vi "FM_Rx_2012_.vi"() -> ()   [LabVIEW 2014]
uses:
  <instrlib>/niUSRP/niUSRP Fetch Rx Data (CDB WDT).vi
  <vilib>/Analysis/3filter.llb/FIR Filter (DBL).vi
  <vilib>/Analysis/3filter.llb/Butterworth Filter (DBL).vi
  <vilib>/Analysis/NI_AALPro.lvlib
  <vilib>/Analysis/NI_AALBase.lvlib
panel:
  out "Demodulated Output":waveform(dbl)(graph)
  in  "stop":bool
  out "error out":errorcluster
  in  "number of samples":i64=200000
  in  "active antenna":string="RX2"
  out "actual gain (dB)":dbl format="%#_6f"
  in  "gain (dB)":dbl format="%#_6f"
  out "actual carrier frequency":dbl=100000.0 format="%#_6p"
  in  "carrier frequency":dbl=915000000.0 format="%#_6p"
  out "actual IQ rate":dbl=100000.0 format="%#_6p"
  in  "IQ rate":dbl=1000000.0 format="%#_6p"
  in  "device names":refnum<k15>="192.168.10.2"
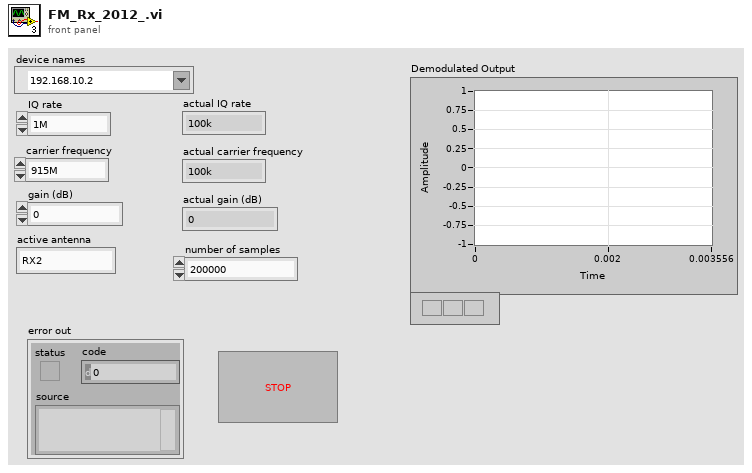
[diagram p1: front panel]
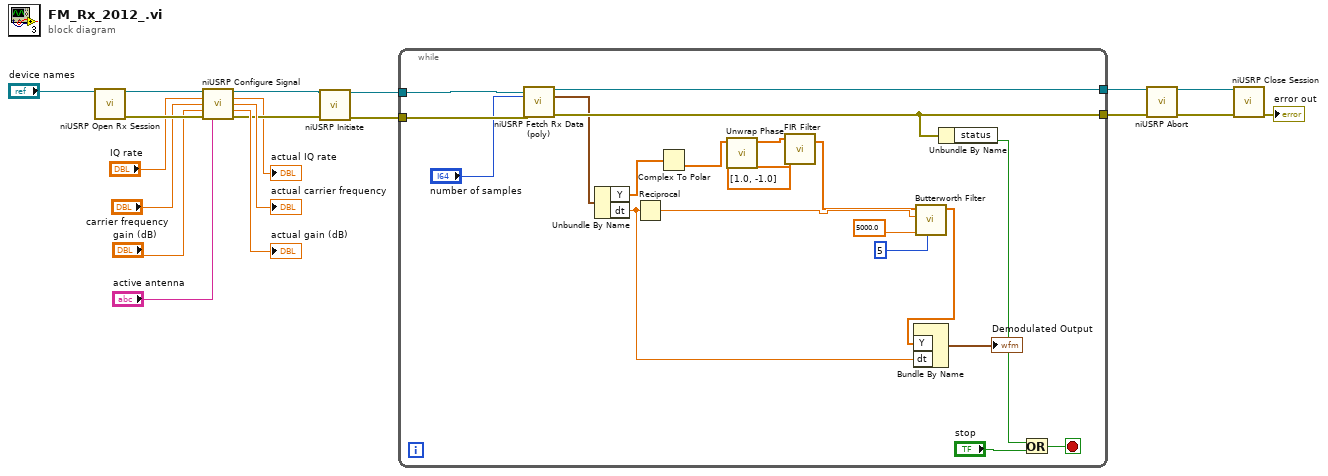
[diagram p0: block diagram]
diagram:
  n1 = call <instrlib>:"niUSRP Open Rx Session.vi"("device names"="device names") -> ("session handle out"=w18:refnum<k15>, "error out"=w17:errorcluster)  [unwired: 13 in]
  n2 = call <instrlib>:"niUSRP Configure Signal.vi"("session handle"=w18, "IQ rate"="IQ rate", "carrier frequency"="carrier frequency", "gain"="gain (dB)", "error in (no error)"=w17, "active antenna"="active antenna") -> ("session handle out"=w11:refnum<k15>, "coerced IQ rate"=→"actual IQ rate":dbl, "coerced carrier frequency"=→"actual carrier frequency":dbl, "coerced gain"=→"actual gain (dB)":dbl, "error out"=w10:errorcluster)  [unwired: 5 in]
  n3 = call <instrlib>:"niUSRP Initiate.vi"("session handle"=w11, "error in (no error)"=w10) -> ("session handle out"=w8:refnum<k15>, "error out"=w7:errorcluster)  [unwired: 12 in]
  n4 = while {
    tunnel: w8 -> [w39]
    tunnel: w7 -> [w38]
    tunnel: [w37] -> w6
    tunnel: [w33] -> w5
    stop <- w36 stop-if-true
    n5 = call-poly <instrlib>:"niUSRP Fetch Rx Data (poly).vi"("session handle"=w39, "number of samples"="number of samples", "error in (no error)"=w38) -> ("session handle out"=w37:refnum<k15>, "data"=w31:waveform(cdb), "error out"=w33:errorcluster)  [unwired: 9 in, 1 out]
    n6 = Unbundle By Name(w31) -> ("Y"=w29:cdb[], "dt"=w26:dbl)
    n7 = Reciprocal(x=w26) -> (1/x=w25:dbl)
    n8 = Complex To Polar(r * e^(i*theta)=w29) -> (theta=w21:dbl[])  [unwired: 1 out]
    n9 = call <vilib>:"Unwrap Phase.vi"("Phase"=w21) -> ("Unwrapped Phase"=w28:dbl[])  [unwired: 9 in, 1 out]
    n10 = call-poly <vilib>:"FIR Filter.vi"("FIR Coefficients"=dbl[] [1.0, -1.0], "X"=w28) -> ("Filtered X"=w24:dbl[])  [unwired: 2 in, 1 out]
    n11 = call-poly <vilib>:"Butterworth Filter.vi"("order"=5, "low cutoff freq: fl"=5000.0 ("high cutoff freq: fh"), "sampling freq: fs"=w25, "X"=w24) -> ("Filtered X"=w22:dbl[])  [unwired: 4 in, 1 out]
    n12 = Bundle By Name("Y"=w22, "dt"=w26) -> (→"Demodulated Output":waveform(dbl))  [unwired: 1 in]
    n13 = Unbundle By Name(w33) -> ("status"=w35:bool)
    n14 = Or(x=w35, y="stop") -> (x .or. y?=w36:bool)
  }
  n15 = call <instrlib>:"niUSRP Abort.vi"("session handle"=w6, "error in (no error)"=w5) -> ("session handle out"=w4:refnum<k15>, "error out"=w3:errorcluster)  [unwired: 12 in]
  n16 = call <instrlib>:"niUSRP Close Session.vi"("session handle"=w4, "error in (no error)"=w3) -> ("error out"=→"error out":errorcluster)  [unwired: 13 in]
